vi "AB_Engine_Check_Excluded_Dep_FileTypes.vi"(9 "exclusionOption":T1, 11 "File":T3) -> (3 "Excluded Dependent File Type?":bool)   [LabVIEW 2020]
uses:
  <vilib>/Utility/lvfile.llb/LVFileType.ctl
  <vilib>/AppBuilder/AB_Exclusion_Option.ctl
  <vilib>/Utility/lvfile.llb/NI_FileType.lvlib
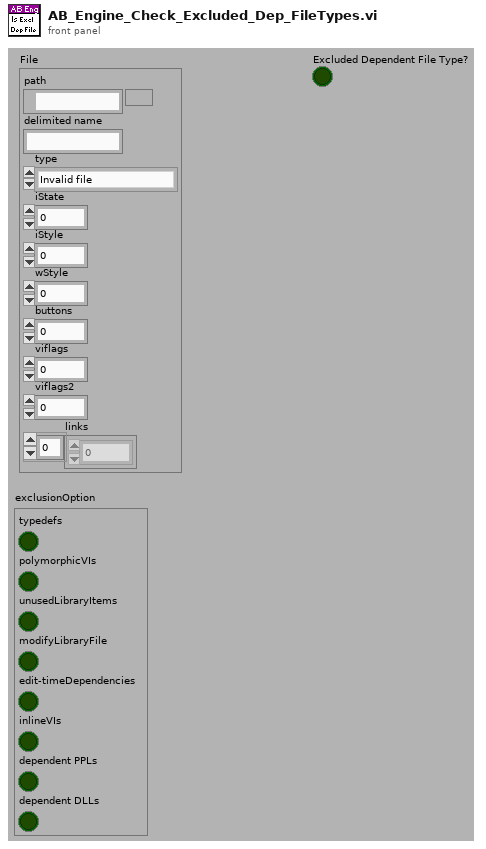
[diagram p1: front panel]
types:
  T1 = typedef "AB_Exclusion_Option.ctl" = cluster{"typedefs":bool, "polymorphicVIs":bool, "unusedLibraryItems":bool, "modifyLibraryFile":bool, "edit-timeDependencies":bool, "inlineVIs":bool, "dependent PPLs":bool, "dependent DLLs":bool}
  T2 = typedef "NI_FileType.lvlib/LVFileType.ctl" = enum32{"Invalid file", "Unknown type", "Instrument", "Control", "Polymorphic VI", "Project", "Library", "LVClass", "XControl", "XNode", "Shared library", ".NET assembly", "ActiveX interface", "CIN", "Run-time menu", "Palette menu", "Help file", "LLB", "XNode Edit Dependency", "Class Private Data Control", "Statechart", "MathScript .m file", "Ladder Diagram", "LVLibp", "XNode Build Dependency"}
  T3 = cluster{"path":path, "delimited name":string, "type":T2, "iState":u32, "iStyle":u16, "wStyle":u16, "buttons":u16, "viflags":u32, "viflags2":u32, "links":u32[]}
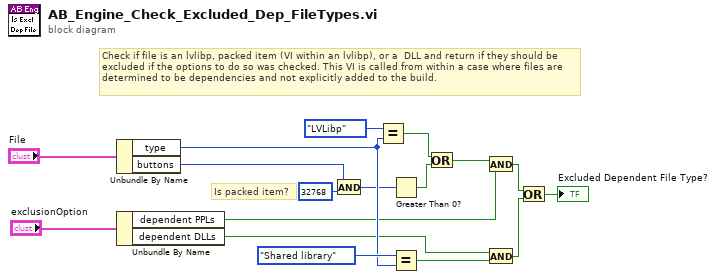
[diagram p0: block diagram]
diagram:
  # "Check if file is an lvlibp, packed item (VI within an lvlibp), or a  DLL and return if they should be excluded if the options to do so was checked. This VI is called from within a case where files are determined to be dependencies and not explicitly added to the build."
  # "Is packed item?"
  n1 = Unbundle By Name("File") -> ("type"=w13:T2, "buttons"=w6:u16)
  n2 = Unbundle By Name("exclusionOption") -> ("dependent PPLs"=w1:bool, "dependent DLLs"=w11:bool)
  n3 = And(x=w6, y=u16 32768) -> (x .and. y?=w5:u16)
  n4 = Equal?(x=LVFileType."LVLibp", y=w13) -> (x = y?=w4:bool)
  n5 = Greater Than 0?(x=w5) -> (x > 0?=w3:bool)
  n6 = Equal?(x=LVFileType."Shared library", y=w13) -> (x = y?=w12:bool)
  n7 = Or(x=w4, y=w3) -> (x .or. y?=w2:bool)
  n8 = And(x=w2, y=w1) -> (x .and. y?=w8:bool)
  n9 = And(x=w11, y=w12) -> (x .and. y?=w9:bool)
  n10 = Or(x=w8, y=w9) -> (x .or. y?=→"Excluded Dependent File Type?":bool)
